vi "Thorlabs-Shut Down MCLS.vi"(7 "ShutDown?":bool, 8 "error in (no error)":errorcluster, 9 "MCSL Controls":T1 {"532"."Power (%)" min=0.0 max=100.0 step=1.0 scale=0.0..100.0; "642"."Power (%)" min=0.0 max=100.0 step=1.0 scale=0.0..100.0; "488"."Power (%)" min=0.0 max=100.0 step=1.0 scale=0.0..100.0; "405"."Power (%)" min=0.0 max=100.0 step=0.1 scale=0.0..100.0}, 10 "Notifiers":T2, 11 "Cluster in":refnum<vi>) -> (0 "error out":errorcluster)   [LabVIEW 2020]
uses:
  _Controls/Notifiers.ctl
  _Controls/MCSL Controls.ctl
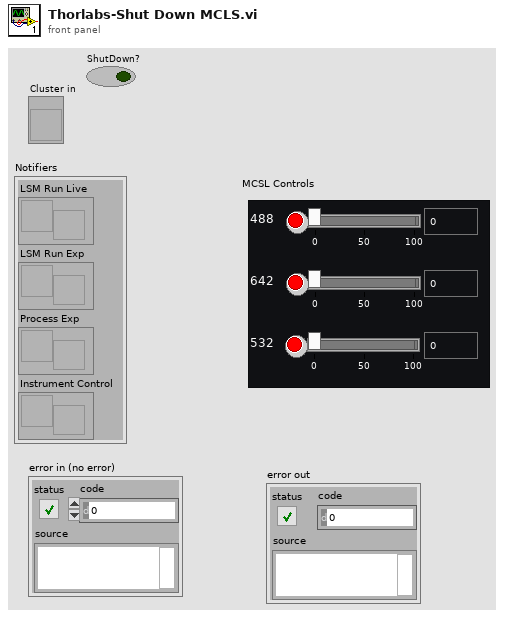
[diagram p1: front panel]
types:
  T1 = typedef "MCSL Controls.ctl" = cluster{"405":cluster{"Enable":bool, "Power (%)":dbl}, "488":cluster{"Enable":bool, "Power (%)":dbl}, "642":cluster{"Enable":bool, "Power (%)":dbl}, "532":cluster{"Enable":bool, "Power (%)":dbl}}
  T2 = typedef "Notifiers.ctl" = cluster{"LSM Run Live":refnum<notifier>, "LSM Run Exp":refnum<notifier>, "Process Exp":refnum<notifier>, "Instrument Control":refnum<notifier>}
  T3 = cluster{"MCSL Controls":T1, "Index of changed laser":i32, "State or Power?":i32}
  T4 = cluster{"notification":string, "Variant":variant}
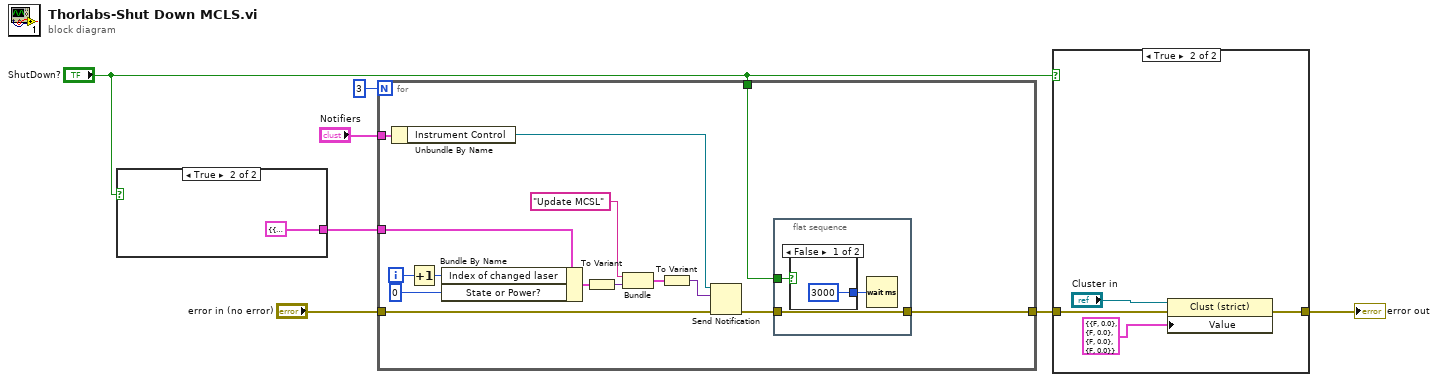
[diagram p0: block diagram]
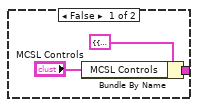
[diagram p3: hidden frame]
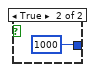
[diagram p4: hidden frame]
diagram:
  n1 = case shown="True" "ShutDown?" {
    tunnel: [w10 T3 {"MCSL Controls"={"405"={"Enable"=FALSE, "Power (%)"=0.0}, "488"={"Enable"=FALSE, "Power (%)"=0.0}, "642"={"Enable"=FALSE, "Power (%)"=0.0}, "532"={"Enable"=FALSE, "Power (%)"=0.0}}, "Index of changed laser"=0, "State or Power?"=0} ("notifier data")] -> w3
    frame False {
      n2 = Bundle By Name(cluster=T3 {"MCSL Controls"={"405"={"Enable"=FALSE, "Power (%)"=0.0}, "488"={"Enable"=FALSE, "Power (%)"=0.0}, "642"={"Enable"=FALSE, "Power (%)"=0.0}, "532"={"Enable"=FALSE, "Power (%)"=0.0}}, "Index of changed laser"=0, "State or Power?"=0} ("notifier data"), "MCSL Controls"="MCSL Controls") -> (w10:T3)
    }
    frame True {
    }
  }
  n3 = for {
    N: 3 -> [_]
    tunnel: "Notifiers" -> [w20]
    tunnel: w3 -> [w13]
    tunnel: "ShutDown?" -> [w12]
    tunnel: "error in (no error)" -> [w21]
    tunnel: [w15] -> w7
    i -> [w18]
    n4 = Unbundle By Name(w20) -> ("Instrument Control"=w26:refnum<notifier>)
    n5 = Increment(x=w18) -> (x+1=w14:i32)
    n6 = Bundle By Name(cluster=w13, "Index of changed laser"=w14, "State or Power?"=0) -> (w19:T3)
    n7 = To Variant(anything=w19) -> (Variant=w22:variant)
    n8 = Bundle("notification"="Update MCSL", "Variant"=w22) -> (w24:T4)  [unwired: 1 in]
    n9 = To Variant(anything=w24) -> (Variant=w23:variant)
    n10 = Send Notification(notification=w23, notifier=w26, error in (no error)=w21) -> (error out=w16:errorcluster)  [unwired: 1 out]
    n11 = flat-sequence {
      tunnel: [w29] -> w15
      tunnel: w16 -> [w29]
      tunnel: w12 -> [w27]
      frame #0 {
        n12 = case shown="False" w27 {
          tunnel: [3000 1000] -> w28
          frame False {
          }
          frame True {
          }
        }
        n13 = Wait (ms)(milliseconds to wait=w28) -> ()  [unwired: 1 out]
      }
    }
  }
  n14 = case shown="True" "ShutDown?" {
    tunnel: w7 -> [w32 w36]
    tunnel: [w32 w34] -> w1
    frame False {
    }
    frame True {
      n15 = property on="Property Node" class="Clust (strict)"(reference="Cluster in", error in=w36, "Value"=T1 {"405"={"Enable"=FALSE, "Power (%)"=0.0}, "488"={"Enable"=FALSE, "Power (%)"=0.0}, "642"={"Enable"=FALSE, "Power (%)"=0.0}, "532"={"Enable"=FALSE, "Power (%)"=0.0}} ("MCSL Controls")) -> (error out=w34:errorcluster)  [unwired: 1 out]
    }
  }
  "error out" <- w1
